vi "Netburner_cntl.vi"() -> ()   [LabVIEW 2013]
panel:
  out "ADC result":string
  out "#  Bytes Read 4":u32
  in  "ADC String  (Chan, #reads)":string="0 1000"
  out "ADC request":string
  out "#  Bytes Read 3":u32
  in  "2nd DAC String  (Chan, Volt)":string="1 -1."
  out "2nd DAC request":string
  out "#  Bytes Read 2":u32
  in  "1st DAC String  (Chan, Volt)":string="0 1"
  out "Error Out":errorcluster={"status"=FALSE, "code"=1073676294, "source"="VISA Read in Netburner_RD.vi->Netburner_cntl.vi"}
  in  "Error In (none)":errorcluster
  out "#  Bytes Read 1":u32
  out "Startup and 1st DAC request":string="\r\n"
  in  "COM Port #":refnum<visa-resource-name>="COM3"
  # "Netburner ADC/DAC Test Interface"
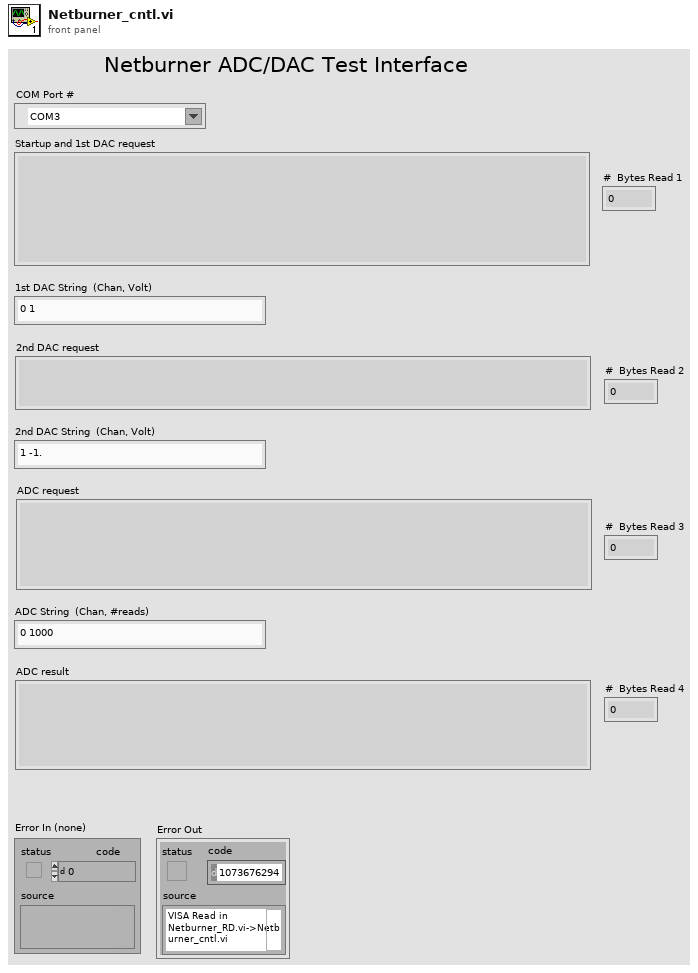
[diagram p1: front panel]
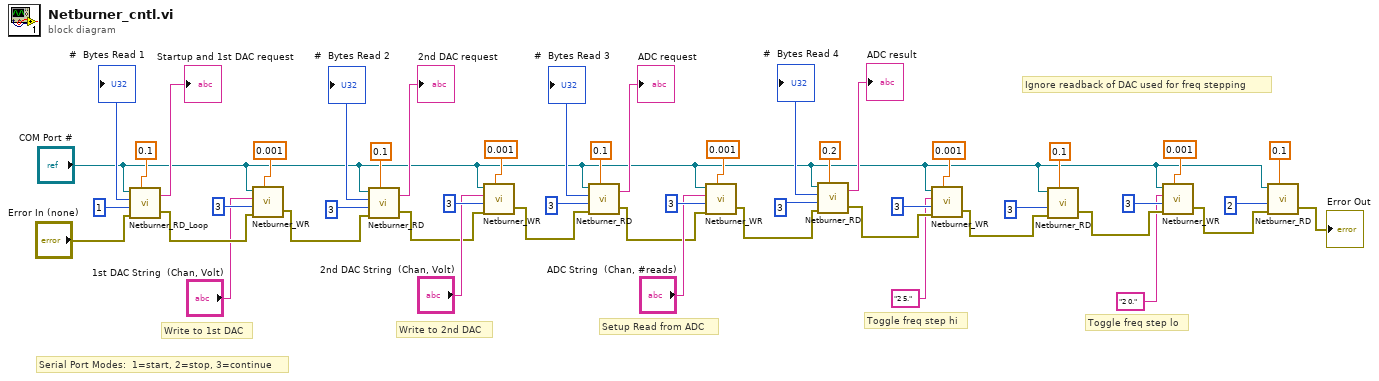
[diagram p0: block diagram]
diagram:
  # "Ignore readback of DAC used for freq stepping"
  # "Serial Port Modes:  1=start, 2=stop, 3=continue"
  # "Toggle freq step lo"
  # "Toggle freq step hi"
  # "Setup Read from ADC"
  # "Write to 2nd DAC"
  # "Write to 1st DAC"
  n1 = call "Netburner_RD_Loop.vi"("VISA resource name (COM Port #)"="COM Port #", "Mode (0)"=1, "Error In (no error)"="Error In (none)", "Wait (sec)"=0.1) -> ("#  Bytes Read"=→"#  Bytes Read 1":u32, "Return String from Device"=→"Startup and 1st DAC request":string, "Error Out"=w44:errorcluster)
  n2 = call "Netburner_WR.vi"("VISA resource name (COM Port #)"="COM Port #", "String to Send"="1st DAC String  (Chan, Volt)", "Mode (0)"=3, "Error In (no error)"=w44, "Wait (sec)"=0.001) -> ("Error Out"=w39:errorcluster)  [unwired: 1 in]
  n3 = call "Netburner_RD.vi"("VISA resource name (COM Port #)"="COM Port #", "Mode (0)"=3, "Error In (no error)"=w39, "Wait (sec)"=0.1) -> ("Number of Bytes Received"=→"#  Bytes Read 2":u32, "Return String from Device"=→"2nd DAC request":string, "Error Out"=w31:errorcluster)
  n4 = call "Netburner_WR.vi"("VISA resource name (COM Port #)"="COM Port #", "String to Send"="2nd DAC String  (Chan, Volt)", "Mode (0)"=3, "Error In (no error)"=w31, "Wait (sec)"=0.001) -> ("Error Out"=w26:errorcluster)  [unwired: 1 in]
  n5 = call "Netburner_RD.vi"("VISA resource name (COM Port #)"="COM Port #", "Mode (0)"=3, "Error In (no error)"=w26, "Wait (sec)"=0.1) -> ("Number of Bytes Received"=→"#  Bytes Read 3":u32, "Return String from Device"=→"ADC request":string, "Error Out"=w22:errorcluster)
  n6 = call "Netburner_WR.vi"("VISA resource name (COM Port #)"="COM Port #", "String to Send"="ADC String  (Chan, #reads)", "Mode (0)"=3, "Error In (no error)"=w22, "Wait (sec)"=0.001) -> ("Error Out"=w17:errorcluster)  [unwired: 1 in]
  n7 = call "Netburner_RD.vi"("VISA resource name (COM Port #)"="COM Port #", "Mode (0)"=3, "Error In (no error)"=w17, "Wait (sec)"=0.2) -> ("Number of Bytes Received"=→"#  Bytes Read 4":u32, "Return String from Device"=→"ADC result":string, "Error Out"=w7:errorcluster)
  n8 = call "Netburner_WR.vi"("VISA resource name (COM Port #)"="COM Port #", "String to Send"="2 5." ("1st DAC String to Send  (Channel, Voltage) 2"), "Mode (0)"=3, "Error In (no error)"=w7, "Wait (sec)"=0.001) -> ("Error Out"=w6:errorcluster)  [unwired: 1 in]
  n9 = call "Netburner_RD.vi"("VISA resource name (COM Port #)"="COM Port #", "Mode (0)"=3, "Error In (no error)"=w6, "Wait (sec)"=0.1) -> ("Error Out"=w5:errorcluster)  [unwired: 2 out]
  n10 = call "Netburner_WR.vi"("VISA resource name (COM Port #)"="COM Port #", "String to Send"="2 0." ("1st DAC String to Send  (Channel, Voltage) 2"), "Mode (0)"=3, "Error In (no error)"=w5, "Wait (sec)"=0.001) -> ("Error Out"=w4:errorcluster)  [unwired: 1 in]
  n11 = call "Netburner_RD.vi"("VISA resource name (COM Port #)"="COM Port #", "Mode (0)"=2, "Error In (no error)"=w4, "Wait (sec)"=0.1) -> ("Error Out"=→"Error Out":errorcluster)  [unwired: 2 out]
